vi "测试-调用Python-只打开一次模型.vi"() -> ()   [LabVIEW 2022 SP3]
panel:
  out "millisecond timer value":u32
  in  "图片路径":string
  in  "图片/视频路径":path
  out "2 error out predict":errorcluster
  out "flag":i32
  out "4 error out object":errorcluster
  out "1 error out ObjInitialize":errorcluster
  out "运行状态":string
  out "return predict":i32
  out "3 error out":errorcluster
  out "appended path":path
  in  "OK Button":bool
  in  "use_gpu":i32
  in  "关闭界面":bool
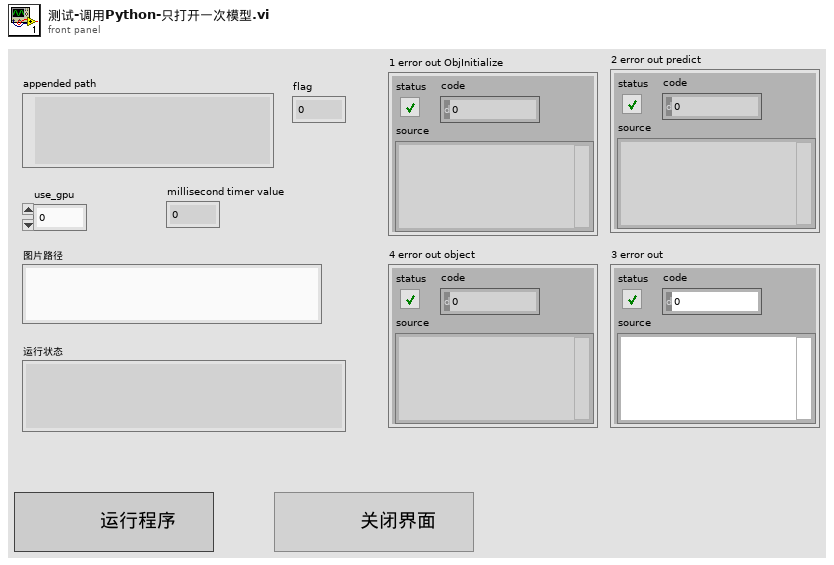
[diagram p1: front panel]
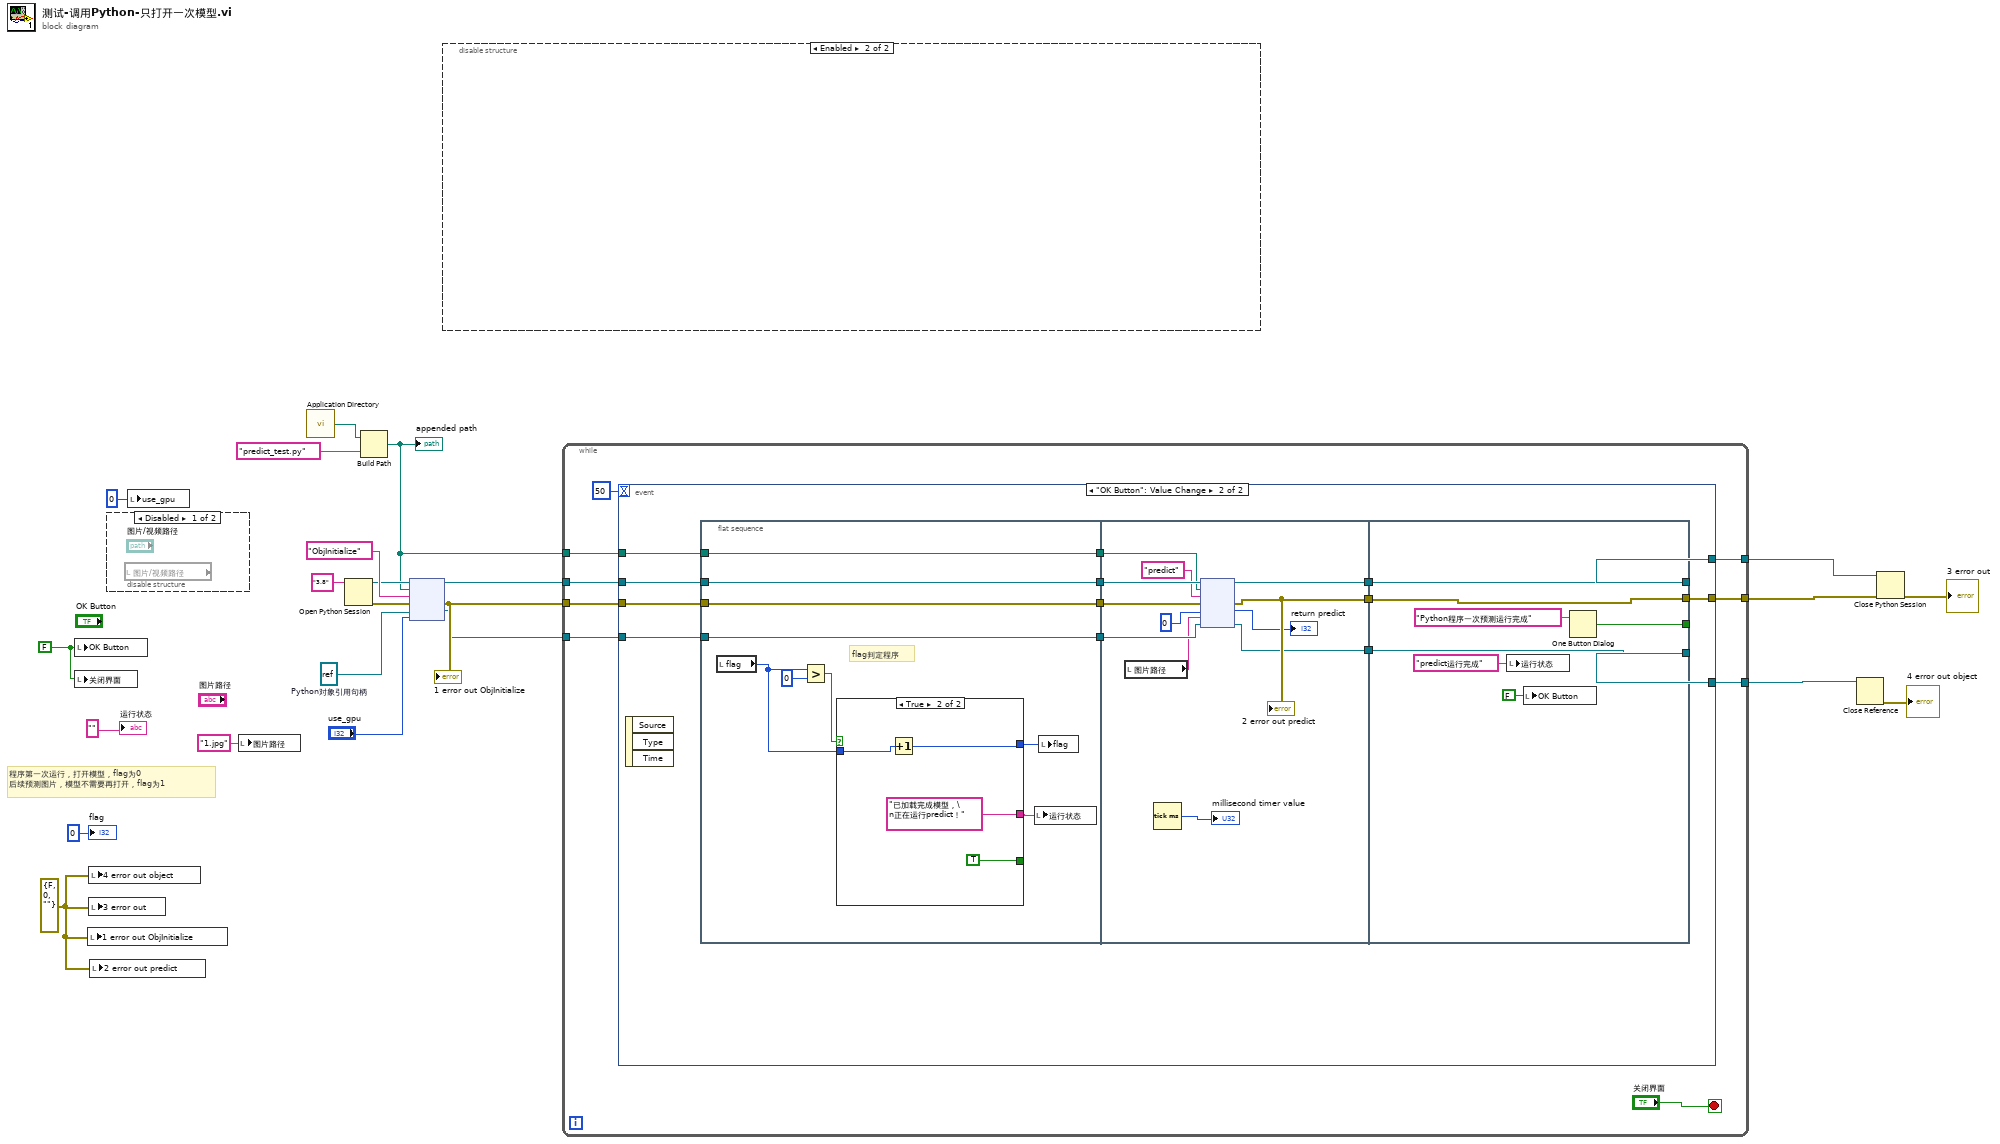
[diagram p0: block diagram]
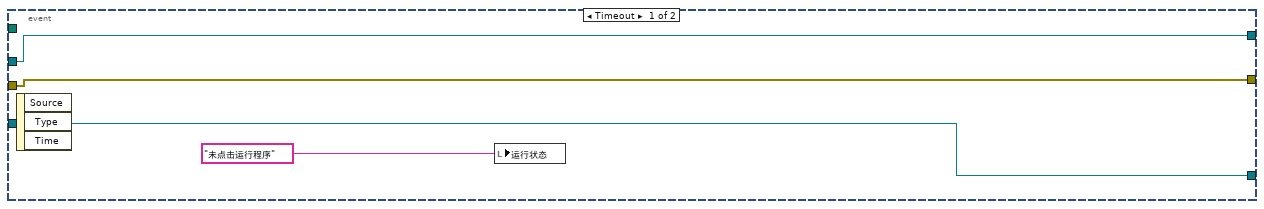
[diagram p3: hidden frame]
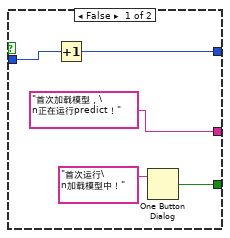
[diagram p4: hidden frame]
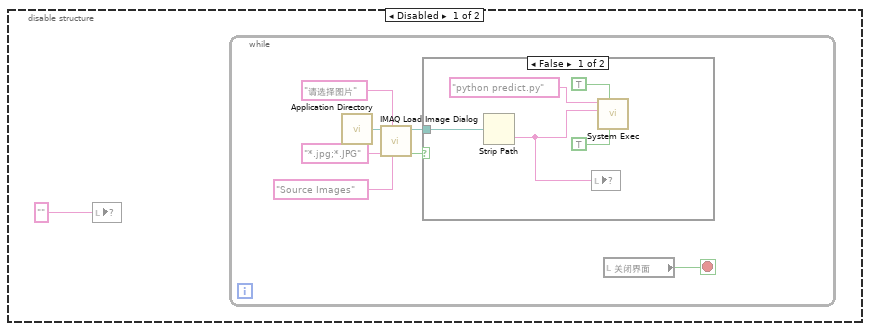
[diagram p5: hidden frame]
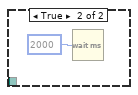
[diagram p6: hidden frame]
diagram:
  w7 = refnum<k38> refnum  # Python对象引用句柄
  w2 = errorcluster {"status"=FALSE, "code"=0, "source"=""} ("error out 2")
  w21 = FALSE ("OK Button")
  # "程序第一次运行，打开模型，flag为0\n后续预测图片，模型不需要再打开，flag为1"
  n1 = local write "OK Button"(w21) -> ()
  n2 = local write "关闭界面"(w21) -> ()
  n3 = local write "1 error out ObjInitialize"(w2) -> ()
  n4 = local write "4 error out object"(w2) -> ()
  n5 = local write "3 error out"(w2) -> ()
  n6 = local write "2 error out predict"(w2) -> ()
  n7 = disable-structure shown="Disabled" {
    frame Disabled {
      n8 = local read "图片/视频路径"() -> ()  [unwired: 1 out]
    }
    frame Enabled {
    }
  }
  n9 = local write "use_gpu"(0 ("use_gpu")) -> ()
  n10 = local write "图片路径"("1.jpg" ("图片路径")) -> ()
  n11 = call <vilib>:"Application Directory.vi"() -> ("Application Directory"=w18:path)
  n12 = Open Python Session(python version="3.8" ("Python version")) -> (session out=w14:refnum<k35>, error out=w15:errorcluster)  [unwired: 2 in]
  n13 = Build Path(base path=w18, name or relative path="predict_test.py" ("名称或相对路径")) -> (appended path=w12:path)
  "appended path" <- w12
  n14 = node(w14, w12, "ObjInitialize" ("函数名称"), w15, w7, "use_gpu") -> (w13:refnum<k35>, w11:errorcluster, w6:refnum<k38>)  [unwired: 1 in, 2 out]
  "1 error out ObjInitialize" <- w11
  n15 = disable-structure shown="Enabled" {
    frame Disabled {
      n16 = local write item#-1("" ("图片/视频路径")) -> ()
      n17 = while {
        stop <- w25 stop-if-true
        n18 = call <vilib>:"Application Directory.vi"() -> ("Application Directory"=w31:path)
        n19 = call "IMAQ Load Image Dialog"("Pattern Label"="Source Images", "Prompt"="请选择图片" ("prompt"), "Pattern"="*.jpg;*.JPG", "Start Path"=w31) -> ("Cancelled?"=w27:bool, "Path"=w26:path)  [unwired: 5 in, 1 out]
        n20 = case shown="False" w27 {
          tunnel: w26 -> [w33 _]
          frame False {
            n21 = Strip Path(path=w33) -> (name=w32:string)  [unwired: 1 out]
            n22 = local write item#-1(w32) -> ()
            n23 = call <vilib>:"System Exec.vi"("run minimized? (F)"=TRUE, "wait until completion? (T)"=TRUE, "standard input"=w32, "command line"="python predict.py") -> ()  [unwired: 4 in, 4 out]
          }
          frame True {
            n24 = Wait (ms)(milliseconds to wait=u32 2000 ("等待时间（毫秒）")) -> ()  [unwired: 1 out]
          }
        }
        n25 = local read "关闭界面"() -> (w25:bool)
      }
    }
    frame Enabled {
    }
  }
  n26 = while {
    tunnel: w13 -> [w45]
    tunnel: w12 -> [w44]
    tunnel: w11 -> [w43]
    tunnel: [w42] -> w10
    tunnel: [w41] -> w9
    tunnel: w6 -> [w39]
    tunnel: [w38] -> w4
    stop <- "关闭界面" stop-if-true
    n27 = event shown="[1] \"OK Button\": Value Change" {
      selector: _ -> [_ _]
      dyn-events: _ -> [_ _]
      timeout: 50 -> [_ _]
      tunnel: w45 -> [w49 w64]
      tunnel: w44 -> [_ w63]
      tunnel: w43 -> [w48 w62]
      tunnel: [w49 w60] -> w42
      tunnel: [w48 w58] -> w41
      tunnel: w39 -> [w47 w57]
      tunnel: [w47 w56] -> w38
      event Timeout {
        n28 = event-data() -> ()  [unwired: 1 in, 3 out]
        n29 = local write "运行状态"("未点击运行程序" ("运行状态")) -> ()
      }
      event "OK Button": Value Change {
        n30 = event-data() -> ()  [unwired: 1 in, 3 out]
        n31 = flat-sequence {
          tunnel: w57 -> [w70]
          tunnel: w62 -> [w71]
          tunnel: w63 -> [w72]
          tunnel: w64 -> [w73]
          tunnel: [w73] -> w54
          tunnel: [w72] -> w53
          tunnel: [w71] -> w52
          tunnel: [w70] -> w51
          tunnel: [w90] -> w61
          tunnel: [w89] -> w59
          tunnel: [w85] -> w55
          tunnel: w54 -> [w94]
          tunnel: w53 -> [w93]
          tunnel: w52 -> [w91]
          tunnel: w51 -> [w86]
          tunnel: [w100] -> _
          tunnel: [w99] -> w60
          tunnel: w61 -> [w99]
          tunnel: w59 -> [w98]
          tunnel: [w98] -> w58
          tunnel: [w95] -> w56
          tunnel: w55 -> [w95]
          frame #0 {
            # "flag判定程序"
            n32 = local read "flag"() -> (w66:i32)
            n33 = Greater?(x=w66, y=0) -> (0:w67:bool)
            n34 = case shown="True" w67 {
              tunnel: ["首次加载模型，\n正在运行predict！" ("运行状态") "已加载完成模型，\n正在运行predict！" ("运行状态")] -> w68
              tunnel: w66 -> [w77 w80]
              tunnel: [w76 w81] -> w65
              tunnel: [w74 TRUE] -> _
              frame False {
                n35 = Increment(x=w77) -> (x+1=w76:i32)
                n36 = One Button Dialog(message="首次运行\n加载模型中！") -> (true=w74:bool)  [unwired: 1 in]
              }
              frame True {
                n37 = Increment(x=w80) -> (x+1=w81:i32)
              }
            }
            n38 = local write "运行状态"(w68) -> ()
            n39 = local write "flag"(w65) -> ()
          }
          frame #1 {
            n40 = local read "图片路径"() -> (w84:string)
            n41 = Tick Count (ms)() -> (millisecond timer value=→"millisecond timer value":u32)
            n42 = node(w94, w93, "predict" ("函数名称"), w91, 0, w84, w86) -> (w90:refnum<k35>, w89:errorcluster, →"return predict":i32, w85:refnum<k38>)  [unwired: 1 in, 2 out]
            "2 error out predict" <- w89
          }
          frame #2 {
            n43 = local write "运行状态"("predict运行完成" ("运行状态")) -> ()
            n44 = local write "OK Button"(FALSE ("OK Button")) -> ()
            n45 = One Button Dialog(message="Python程序一次预测运行完成") -> (true=w100:bool)  [unwired: 1 in]
          }
        }
      }
    }
  }
  n46 = Close Reference(reference=w4) -> (error out=→"4 error out object":errorcluster)  [unwired: 1 in]
  n47 = Close Python Session(session in=w10, error in=w9) -> (11:→"3 error out":errorcluster)
  "运行状态" <- ""
  "flag" <- 0
